vi "Main Photon Focus.vi"() -> ()   [LabVIEW 2021]
uses:
  <vilib>/vision/driver/NI_Vision_Acquisition_Software.lvlib
  <resource>/objmgr/imaqdx.rc
panel:
  out "Image":T1(plugin-control)
  in  "Camera Name":refnum<k21> caption="IMAQdx Session"
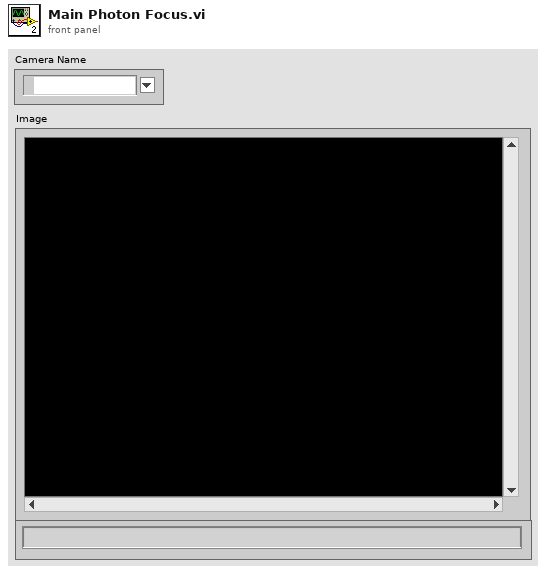
[diagram p1: front panel]
types:
  T1 = typedef "IMAQ Image.ctl" = refnum<image>
  T2 = typedef "Image Type" = u32
  T3 = typedef "IMAQdx.ctl" = refnum<k21>
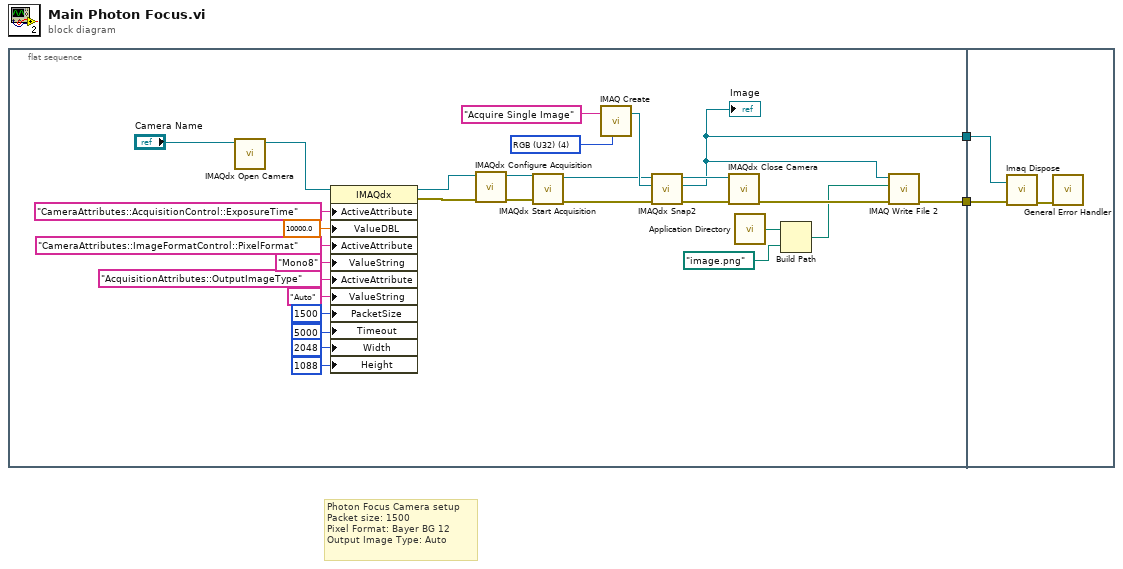
[diagram p0: block diagram]
diagram:
  # "Photon Focus Camera setup\nPacket size: 1500\nPixel Format: Bayer BG 12\nOutput Image Type: Auto"
  n1 = flat-sequence {
    tunnel: [w24] -> w2
    tunnel: [w26] -> w1
    tunnel: w2 -> [w34]
    tunnel: w1 -> [w33]
    frame #0 {
      w27 = T2 4 items=["Grayscale (U8)", "Grayscale (I16)", "Grayscale (SGL)", "Complex (CSG)", "RGB (U32)", "HSL (U32)", "RGB (U64)", "Grayscale (U16)"] ("Image Type")
      n2 = call <vilib>:"IMAQdx Open Camera.vi"("Session In"="Camera Name") -> ("Session Out"=w15:T3)  [unwired: 2 in, 8 out]
      n3 = property class="IMAQdx"(reference=w15, "ActiveAttribute"="CameraAttributes::AcquisitionControl::ExposureTime", "ValueDBL"=10000.0, "ActiveAttribute"="CameraAttributes::ImageFormatControl::PixelFormat", "ValueString"="Mono8", "ActiveAttribute"="AcquisitionAttributes::OutputImageType", "ValueString"="Auto", "PacketSize"=u32 1500, "Timeout"=u32 5000, "Width"=u32 2048, "Height"=u32 1088) -> (reference out=w14:T3, error out=w11:errorcluster)  [unwired: 1 in]
      n4 = call <vilib>:"IMAQdx Configure Acquisition.vi"("error in"=w11, "Session In"=w14) -> ("error out"=w12:errorcluster, "Session Out"=w13:T3)  [unwired: 8 in]
      n5 = call <vilib>:"IMAQdx Start Acquisition.vi"("error in"=w12, "Session In"=w13) -> ("error out"=w10:errorcluster, "Session Out"=w9:T3)  [unwired: 8 in]
      n6 = call "IMAQ Create"("Image Name"="Acquire Single Image", "Image Type"=w27) -> ("New Image"=w29:T1)  [unwired: 2 in, 2 out]
      n7 = call <vilib>:"IMAQdx Snap2.vi"("error in"=w10, "Image In"=w29, "Session In"=w9) -> ("error out"=w30:errorcluster, "Image Out"=w26:T1, "Session Out"=w31:T3)  [unwired: 6 in]
      "Image" <- w26
      n8 = call <vilib>:"IMAQdx Close Camera.vi"("error in"=w30, "Session In"=w31) -> ("error out"=w25:errorcluster)  [unwired: 9 out]
      n9 = call <vilib>:"Application Directory.vi"() -> ("Application Directory"=w23:path)
      n10 = Build Path(base path=w23, name or relative path=path "image.png") -> (appended path=w22:path)
      n11 = call-poly "IMAQ Write File 2"("error in (no error)"=w25, "File Path"=w22, "Image"=w26) -> ("error out"=w24:errorcluster)  [unwired: 7 in, 1 out]
    }
    frame #1 {
      n12 = call "Imaq Dispose"("Image"=w33, "error in (no error)"=w34) -> ("error out"=w32:errorcluster)  [unwired: 4 in]
      n13 = call <vilib>:"General Error Handler.vi"("error in (no error)"=w32) -> ()  [unwired: 2 in, 13 out]
    }
  }
